vi "RSZVB Set IF Gain.vi"(7 "IF Gain (0: Auto)":i32(ring) items=["Auto", "Low Noise", "Low Distortion"], 8 "error in (no error)":errorcluster {"code" format="%.0x"}, 9 "Port (1)":i32=1, 10 "Channel (1)":i32=1, 11 "VISA session":refnum<visa-resource-name>) -> (0 "error out":errorcluster {"code" format="%.0x"}, 3 "dup VISA session":refnum<visa-resource-name>)   [LabVIEW 2011]
doc: "This VI selects the IF gain in the measurement channel b. \n\nRemote-control command(s):\n[SENSe<Ch>:]POWer:IFGain<Pt>:MEASure AUTO | LNOise | LDIStortion"
uses:
  _utility/RSZVB Global Data.vi
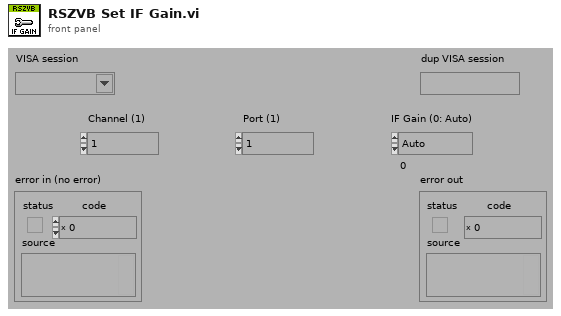
[diagram p1: front panel]
types:
  T1 = cluster{"Error Checking (T: On)":bool, "Installed Options":string[], "Data Valid?":bool, "Ports":i32, "Model":string[], "Option Checking (T: On)":bool}[]
  T2 = cluster{"Error Checking (T: On)":bool, "Installed Options":string[], "Data Valid?":bool, "Ports":i32, "Model":string[], "Option Checking (T: On)":bool}
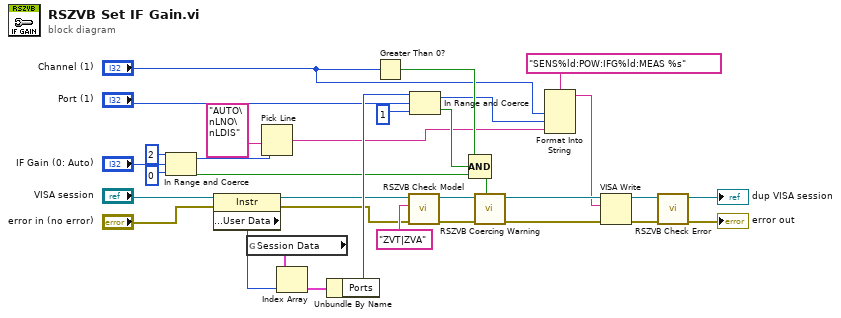
[diagram p0: block diagram]
diagram:
  n1 = In Range and Coerce(upper limit=2 ("lower limit"), x="IF Gain (0: Auto)", lower limit=0) -> (coerced(x)=w9:i32, In Range?=w8:bool)
  n2 = property class="Instr"(reference="VISA session", error in="error in (no error)") -> (reference out=w2:refnum<visa-resource-name>, error out=w1:errorcluster, "General Settings:User Data"=w22:u32)
  n3 = global read "RSZVB Global Data.vi" "Session Data"() -> (w23:T1)
  n4 = Pick Line(multi-line string="AUTO\nLNO\nLDIS", line index=w9) -> (output string=w6:string)  [unwired: 1 in]
  n5 = Index Array(array=w23, index=w22) -> (element=w24:T2)
  n6 = Unbundle By Name(w24) -> ("Ports"=w21:i32)
  n7 = Greater Than 0?(x="Channel (1)") -> (x > 0?=w25:bool)
  n8 = call "RSZVB Check Model.vi"("error in (no error)"=w1, "Model"="ZVT|ZVA" ("Options"), "VISA session"=w2) -> ("error out"=w4:errorcluster, "dup VISA session"=w3:refnum<visa-resource-name>)  [unwired: 7 in]
  n9 = In Range and Coerce(upper limit=w21, x="Port (1)", lower limit=1) -> (coerced(x)=w19:i32, In Range?=w20:bool)
  n10 = Compound Arithmetic op=AND(w25, w20, w8) -> (w27:bool)
  n11 = call "RSZVB Coercing Warning.vi"("In Range?"=w27, "error in (no error)"=w4, "VISA session"=w3) -> ("error out"=w30:errorcluster, "dup VISA session"=w31:refnum<visa-resource-name>)  [unwired: 7 in]
  n12 = Format Into String(format string="SENS%ld:POW:IFG%ld:MEAS %s", "Channel (1)", w19, w6) -> (resulting string=w26:string)  [unwired: 2 in, 1 out]
  n13 = VISA Write(VISA resource name=w31, write buffer=w26, error in (no error)=w30) -> (VISA resource name out=w28:refnum<visa-resource-name>, error out=w29:errorcluster)  [unwired: 1 out]
  n14 = call "RSZVB Check Error.vi"("error in (no error)"=w29, "VISA session"=w28) -> ("error out"=→"error out":errorcluster, "dup VISA session"=→"dup VISA session":refnum<visa-resource-name>)  [unwired: 8 in]
